vi "Zadanie4.vi"() -> ()   [LabVIEW 2011]
panel:
  out "Waveform Chart":dbl(graph)
  in  "Выбор сигнала":bool
  in  "stop":bool
  out "Numeric":u32
  # "Случ. числа"
  # "Синусоида"
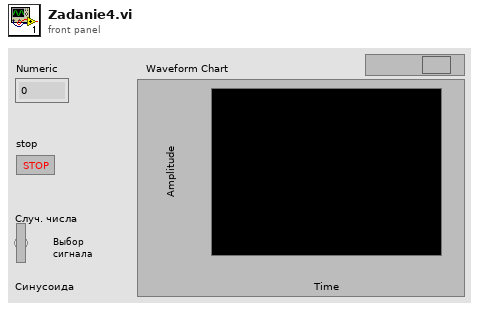
[diagram p1: front panel]
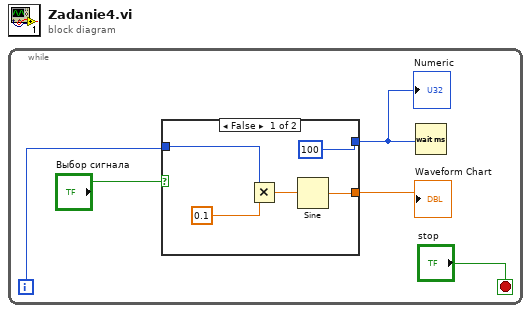
[diagram p0: block diagram]
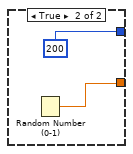
[diagram p2: hidden frame]
diagram:
  n1 = while {
    i -> [w2]
    stop <- "stop" stop-if-true
    n2 = case shown="False" "Выбор сигнала" {
      tunnel: [w9 w12] -> w4
      tunnel: [u32 100 u32 200] -> w3
      tunnel: w2 -> [w6 _]
      frame False {
        n3 = Multiply(x=w6, y=0.1) -> (x*y=w8:dbl)
        n4 = Sine(x=w8) -> (sin(x)=w9:dbl)
      }
      frame True {
        n5 = Random Number (0-1)() -> (number: 0 to 1=w12:dbl)
      }
    }
    "Numeric" <- w3
    "Waveform Chart" <- w4
    n6 = Wait (ms)(milliseconds to wait=w3) -> ()  [unwired: 1 out]
  }
